vi "TempMonitor_Command_Enumerations.vi"() -> ()   [LabVIEW 2012]
panel:
  in  "TEMP ALERT NOTIFICATION INTERVAL (ms)":u32=1000
  in  "Delimiter":string
  in  "TEMP TEXT LENGTH":u8=56
  in  "TEMP CHECK INTERVAL (ms)":u32=1000
  in  "TEMP RESOLUTION (C)":dbl=1.0
  in  "ALERT_TEMP_OUTSIDE_LIMITS":u16=64
  in  "CMD_RESPOND_HIGH_LIMIT":u16=63
  in  "CMD_RESPOND_LOW_LIMIT":u16=62
  in  "CMD_REQUEST_HIGH_LIMIT":u16=61
  in  "CMD_REQUEST_LOW_LIMIT":u16=60
  in  "CMD_SET_HIGH_LIMIT":u16=59
  in  "CMD_SET_LOW_LIMIT":u16=58
  in  "CMD_RESPOND_TEMP":u16=57
  in  "CMD_REQUEST_TEMP":u16=56
  # "COMMAND ENUMERATIONS"
  # "CONSTANTS"
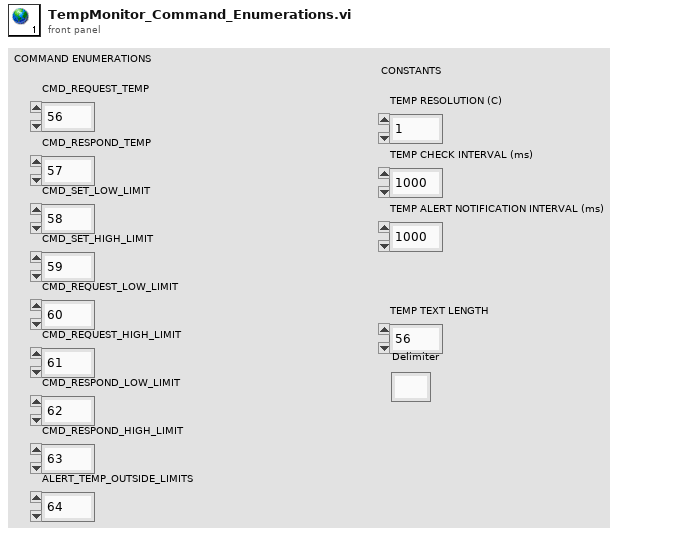
[diagram p1: front panel]
diagram:
